vi "SubVI_Amplifier_Setup_EEG_Acc.vi"(7 "LINX Resource in":T1, 8 "error in (no error)":errorcluster, 9 "Size of Rows for EEG Setup":u8[](array[numeric]), 10 "Amplifier Acc Setup":u8[][](array[numeric]), 11 "Amplifier EEG Setup":u8[][](array[numeric])) -> (0 "error out":errorcluster, 3 "LINX Resource out":T1)   [LabVIEW 2020]
uses:
  <vilib>/MakerHub/LINX/Private/Type Defs/LINX Ref.ctl
  <vilib>/MakerHub/LINX/Private/Type Defs/Platform.ctl
  <vilib>/MakerHub/LINX/Private/Type Defs/Interface.ctl
  <vilib>/MakerHub/LINX/Private/Device/Type Defs/LINX Device Config.ctl
  <vilib>/MakerHub/LINX/Private/Device/Type Defs/TCP Config.ctl
  <vilib>/MakerHub/LINX/Private/Device/Type Defs/Channels.ctl
  <vilib>/MakerHub/LINX/Private/Type Defs/Peripherals/SPI/SPI Configuration.ctl
  <vilib>/MakerHub/LINX/Private/Type Defs/Peripherals/SPI/SPI Bit Order.ctl
  <vilib>/MakerHub/LINX/Private/Type Defs/Peripherals/SPI/SPI Mode.ctl
  <vilib>/MakerHub/LINX/Public/Peripherals/SPI/SPI CS Config.ctl
  <vilib>/MakerHub/LINX/Private/Type Defs/Peripherals/SPI/SPI CS Logic Level.ctl
  <vilib>/MakerHub/LINX/Public/Peripherals/Digital/Digital Write 1 Chan.vi
  <vilib>/MakerHub/LINX/Public/Peripherals/Digital/Digital Read 1 Chan.vi
  <vilib>/MakerHub/LINX/Public/Peripherals/SPI/SPI Write Read N Frames.vi
  <vilib>/MakerHub/LINX/Public/Peripherals/Digital/Digital Write N Chans.vi
  <vilib>/MakerHub/LINX/Public/Peripherals/Digital/Digital Read N Chans.vi
  <vilib>/MakerHub/LINX/Private/Local IO/LinxSpiWriteRead.vi
  <vilib>/MakerHub/LINX/Public/Utilities/Check Channel.vi
  <vilib>/MakerHub/LINX/Private/Local IO/LinxDigitalWrite.vi
  <vilib>/MakerHub/LINX/Private/Local IO/LinxDigitalRead.vi
  <vilib>/MakerHub/LINX/Private/Local IO/Handle Errors.vi
  <vilib>/MakerHub/LINX/Private/Utilties/Generate Error.vi
  Global 1.vi
  <vilib>/MakerHub/LINX/LMH-LINX.lvlib
  <vilib>/MakerHub/LINX/Private/Device/Device.lvlib
panel:
  out "Read Data":u8[](array[numeric])
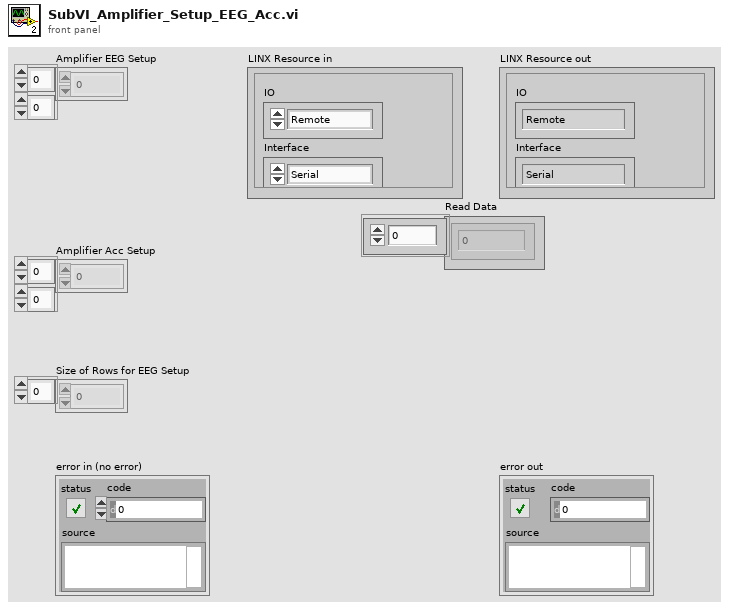
[diagram p1: front panel]
types:
  T1 = typedef "LMH-LINX.lvlib/LINX Ref.ctl" = cluster{"IO":T2, "Interface":T3, "LINX Device Config":T4}
  T2 = typedef "LMH-LINX.lvlib/Platform.ctl" = enum16{"Remote", "Local"}
  T3 = typedef "LMH-LINX.lvlib/Interface.ctl" = enum16{"Serial", "TCP"}
  T4 = typedef "LMH-LINX.lvlib/Device.lvlib/LINX Device Config.ctl" = cluster{"Interface":T3, "COM Port":refnum<visa-resource-name>, "TCP Configuration":T5, "Device Family":u8, "Device ID":u8, "Device Name":string, "TCP Ref":refnum<k5>, "Channels":T6}
  T5 = typedef "LMH-LINX.lvlib/Device.lvlib/TCP Config.ctl" = cluster{"IP Address":string, "Port":u16}
  T6 = typedef "LMH-LINX.lvlib/Channels.ctl" = cluster{"DI":u8[], "DO":u8[], "AI":u8[], "AO":u8[], "PWM":u8[], "QE":u8[], "UART":u8[], "I2C 2":u8[], "SPI":u8[], "CAN":u8[], "Servo":u8[], "AI Ref (V)":dbl, "AI Resolution (Bits)":u8, "AO Ref (V)":dbl, "AO Resolution (Bits)":u8}
  T7 = typedef "LMH-LINX.lvlib/SPI CS Config.ctl" = cluster{"CS Channel":u8, "CS Logic Level":T8}
  T8 = typedef "LMH-LINX.lvlib/SPI CS Logic Level.ctl" = enum8{"Active Low", "Active High"}
  T9 = typedef "LMH-LINX.lvlib/SPI Configuration.ctl" = cluster{"Clock Frequency":u32, "Bit Order":T10, "SPI Mode":T11}
  T10 = typedef "LMH-LINX.lvlib/SPI Bit Order.ctl" = enum8{"LSb First", "MSb First"}
  T11 = typedef "LMH-LINX.lvlib/SPI Mode.ctl" = enum8{"Mode 0", "Mode 1", "Mode 2", "Mode 3"}
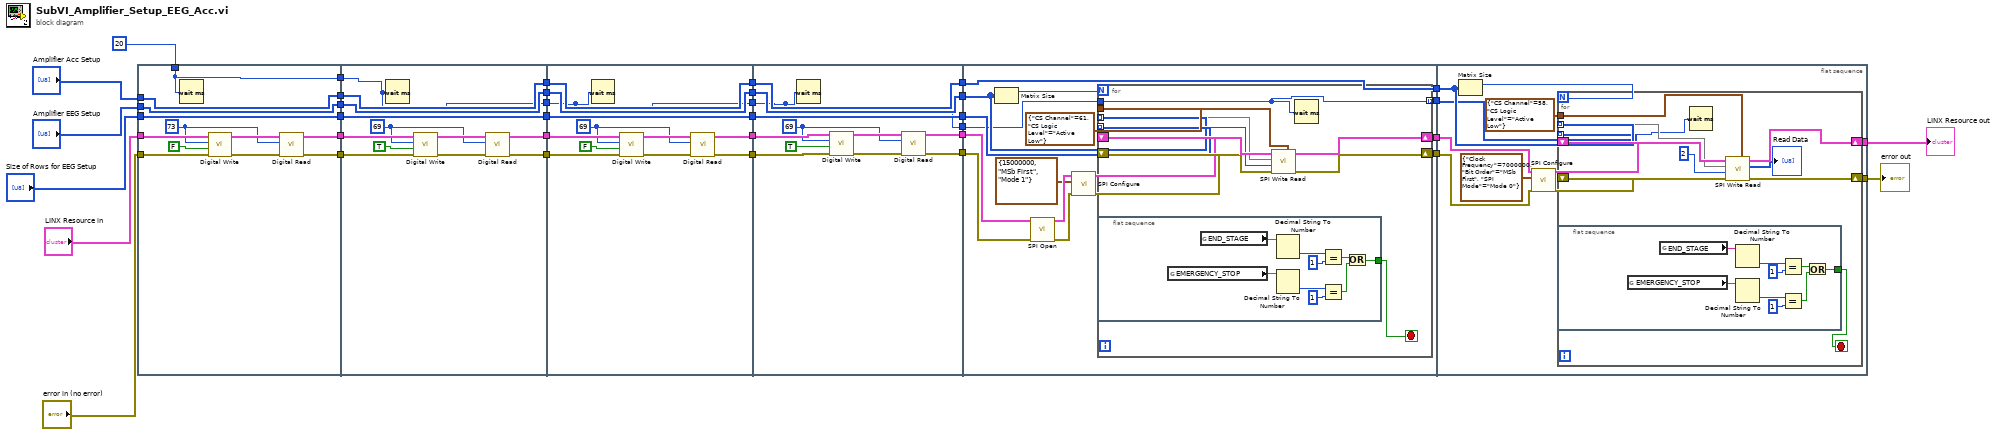
[diagram p0: block diagram]
diagram:
  n1 = flat-sequence {
    tunnel: "error in (no error)" -> [w47]
    tunnel: "LINX Resource in" -> [w46]
    tunnel: "Amplifier EEG Setup" -> [w40]
    tunnel: [w40] -> w29
    tunnel: "Size of Rows for EEG Setup" -> [w39]
    tunnel: [w39] -> w28
    tunnel: "Amplifier Acc Setup" -> [w38]
    tunnel: [w38] -> w27
    tunnel: [w43] -> w26
    tunnel: [w42] -> w25
    tunnel: u32 20 ("milliseconds to wait") -> [w37]
    tunnel: [w37] -> w5
    tunnel: w29 -> [w52]
    tunnel: [w52] -> w24
    tunnel: w28 -> [w51]
    tunnel: [w51] -> w23
    tunnel: w27 -> [w50]
    tunnel: [w50] -> w22
    tunnel: w26 -> [w60]
    tunnel: w25 -> [w59]
    tunnel: [w54] -> w21
    tunnel: [w53] -> w20
    tunnel: w5 -> [w49]
    tunnel: [w49] -> w4
    tunnel: w24 -> [w64]
    tunnel: [w64] -> w19
    tunnel: w23 -> [w63]
    tunnel: [w63] -> w18
    tunnel: w22 -> [w62]
    tunnel: [w62] -> w17
    tunnel: w21 -> [w71]
    tunnel: w20 -> [w70]
    tunnel: [w66] -> w16
    tunnel: [w67] -> w15
    tunnel: w4 -> [w61]
    tunnel: [w61] -> w3
    tunnel: w19 -> [w76]
    tunnel: [w76] -> w14
    tunnel: w18 -> [w75]
    tunnel: [w75] -> w13
    tunnel: w17 -> [w74]
    tunnel: [w74] -> w12
    tunnel: w16 -> [w83]
    tunnel: w15 -> [w82]
    tunnel: [w79] -> w11
    tunnel: [w78] -> w10
    tunnel: w3 -> [w73]
    tunnel: [w73] -> w2
    tunnel: w14 -> [w88]
    tunnel: w13 -> [w90]
    tunnel: w12 -> [w87]
    tunnel: [w87] -> w9
    tunnel: w11 -> [w96]
    tunnel: w10 -> [w97]
    tunnel: [w94] -> w8
    tunnel: [w93] -> w7
    tunnel: w2 -> [w86]
    tunnel: [w85] -> w1
    tunnel: w9 -> [w124]
    tunnel: [w121] -> w33
    tunnel: [w120] -> w34
    tunnel: w8 -> [w122]
    tunnel: w7 -> [w123]
    tunnel: w1 -> [w119]
    frame #0 {
      w41 = u8 73 ("DO Channel")
      n2 = Wait (ms)(milliseconds to wait=w37) -> ()  [unwired: 1 out]
      n3 = call-poly <vilib>:"Digital Write.vi"("Error In"=w47, "Output Value"=FALSE, "DO Channel"=w41, "LINX Resource"=w46) -> ("Error Out"=w45:errorcluster, "LINX Resource"=w44:T1)  [unwired: 6 in]
      n4 = call-poly <vilib>:"Digital Read.vi"("Error In"=w45, "DI Channel"=w41, "LINX Resource"=w44) -> ("Error Out"=w42:errorcluster, "LINX Resource"=w43:T1)  [unwired: 6 in, 1 out]
    }
    frame #1 {
      w55 = u8 69 ("DO Channel")
      n5 = Wait (ms)(milliseconds to wait=w49) -> ()  [unwired: 1 out]
      n6 = call-poly <vilib>:"Digital Write.vi"("Error In"=w59, "Output Value"=TRUE, "DO Channel"=w55, "LINX Resource"=w60) -> ("Error Out"=w57:errorcluster, "LINX Resource"=w56:T1)  [unwired: 6 in]
      n7 = call-poly <vilib>:"Digital Read.vi"("Error In"=w57, "DI Channel"=w55, "LINX Resource"=w56) -> ("Error Out"=w53:errorcluster, "LINX Resource"=w54:T1)  [unwired: 6 in, 1 out]
    }
    frame #2 {
      w65 = u8 69 ("DO Channel")
      n8 = Wait (ms)(milliseconds to wait=w61) -> ()  [unwired: 1 out]
      n9 = call-poly <vilib>:"Digital Write.vi"("Error In"=w70, "Output Value"=FALSE, "DO Channel"=w65, "LINX Resource"=w71) -> ("Error Out"=w69:errorcluster, "LINX Resource"=w68:T1)  [unwired: 6 in]
      n10 = call-poly <vilib>:"Digital Read.vi"("Error In"=w69, "DI Channel"=w65, "LINX Resource"=w68) -> ("Error Out"=w67:errorcluster, "LINX Resource"=w66:T1)  [unwired: 6 in, 1 out]
    }
    frame #3 {
      w77 = u8 69 ("DO Channel")
      n11 = Wait (ms)(milliseconds to wait=w73) -> ()  [unwired: 1 out]
      n12 = call-poly <vilib>:"Digital Write.vi"("Error In"=w82, "Output Value"=TRUE, "DO Channel"=w77, "LINX Resource"=w83) -> ("Error Out"=w81:errorcluster, "LINX Resource"=w80:T1)  [unwired: 6 in]
      n13 = call-poly <vilib>:"Digital Read.vi"("Error In"=w81, "DI Channel"=w77, "LINX Resource"=w80) -> ("Error Out"=w78:errorcluster, "LINX Resource"=w79:T1)  [unwired: 6 in, 1 out]
    }
    frame #4 {
      n14 = Matrix Size(0:w88) -> (1:w89:i32)  [unwired: 1 out]
      n15 = call <vilib>:"SPI Open.vi"("Error In"=w97, "LINX Resource"=w96) -> ("Error Out"=w99:errorcluster, "LINX Resource"=w100:T1)  [unwired: 8 in]
      n16 = call <vilib>:"SPI Configure.vi"("Error In"=w99, "SPI Configuration"=T9 {"Clock Frequency"=15000000, "Bit Order"=enum."MSb First", "SPI Mode"=enum."Mode 1"}, "LINX Resource"=w100) -> ("Error Out"=w92:errorcluster, "LINX Resource"=w91:T1)  [unwired: 6 in, 1 out]
      n17 = for {
        N: w89 -> [_]
        shift-right: [w107] -> w94
        shift-left: w91 -> [w109]
        shift-right: [w106] -> w93
        shift-left: w92 -> [w108]
        tunnel: w90 -> [w104] mode=indexing
        tunnel: w88 -> [w105] mode=indexing
        tunnel: T7 {"CS Channel"=61, "CS Logic Level"=enum."Active Low"} ("CS Configuration") -> [w103]
        tunnel: w86 -> [w102]
        tunnel: [w102] -> w85 mode=indexing
        stop <- w101 stop-if-true
        n18 = flat-sequence {
          tunnel: [w110] -> w101
          frame #0 {
            n19 = global read "Global 1.vi" "EMERGENCY_STOP"() -> (w113:string)
            n20 = global read "Global 1.vi" "END_STAGE"() -> (w118:string)
            n21 = Decimal String To Number(string=w118) -> (number=w117:i32)  [unwired: 2 in, 1 out]
            n22 = Decimal String To Number(string=w113) -> (number=w115:i32)  [unwired: 2 in, 1 out]
            n23 = Equal?(x=w117, y=1) -> (x = y?=w111:bool)
            n24 = Equal?(x=w115, y=1) -> (x = y?=w112:bool)
            n25 = Or(x=w111, y=w112) -> (x .or. y?=w110:bool)
          }
        }
        n26 = call-poly <vilib>:"SPI Write Read.vi"("CS Configuration"=w103, "Error In"=w108, "SPI Frame Size"=w104, "Data"=w105, "LINX Resource"=w109) -> ("Error Out"=w106:errorcluster, "LINX Resource"=w107:T1)  [unwired: 3 in, 2 out]
        n27 = Wait (ms)(milliseconds to wait=w102) -> ()  [unwired: 1 out]
      }
    }
    frame #5 {
      n28 = Matrix Size(0:w124) -> (1:w129:i32)  [unwired: 1 out]
      n29 = call <vilib>:"SPI Configure.vi"("Error In"=w123, "SPI Configuration"=T9 {"Clock Frequency"=7000000, "Bit Order"=enum."MSb First", "SPI Mode"=enum."Mode 0"}, "LINX Resource"=w122) -> ("Error Out"=w127:errorcluster, "LINX Resource"=w128:T1)  [unwired: 6 in, 1 out]
      n30 = for {
        N: w129 -> [_]
        shift-right: [w137] -> w120
        shift-left: w128 -> [w139]
        shift-right: [w136] -> w121
        shift-left: w127 -> [w138]
        tunnel: w124 -> [w135] mode=indexing
        tunnel: T7 {"CS Channel"=58, "CS Logic Level"=enum."Active Low"} ("CS Configuration") -> [w134]
        tunnel: w119 -> [w131] mode=indexing
        stop <- w130 stop-if-true
        n31 = flat-sequence {
          tunnel: [w140] -> w130
          frame #0 {
            n32 = global read "Global 1.vi" "EMERGENCY_STOP"() -> (w143:string)
            n33 = global read "Global 1.vi" "END_STAGE"() -> (w148:string)
            n34 = Decimal String To Number(string=w148) -> (number=w147:i32)  [unwired: 2 in, 1 out]
            n35 = Decimal String To Number(string=w143) -> (number=w145:i32)  [unwired: 2 in, 1 out]
            n36 = Equal?(x=w147, y=1) -> (x = y?=w141:bool)
            n37 = Equal?(x=w145, y=1) -> (x = y?=w142:bool)
            n38 = Or(x=w141, y=w142) -> (x .or. y?=w140:bool)
          }
        }
        n39 = Wait (ms)(milliseconds to wait=w131) -> ()  [unwired: 1 out]
        n40 = call-poly <vilib>:"SPI Write Read.vi"("CS Configuration"=w134, "Error In"=w138, "SPI Frame Size"=u8 2, "Data"=w135, "LINX Resource"=w139) -> ("Error Out"=w136:errorcluster, "Read Data"=→"Read Data":u8[], "LINX Resource"=w137:T1)  [unwired: 3 in, 1 out]
      }
    }
  }
  "LINX Resource out" <- w34
  "error out" <- w33
